vi "Erode_Low_Manual.vi"(4 "Error IN Toolkit":i32, 5 "Error IN LabVIEW":errorcluster, 6 "Radio":i32, 8 "Blocks":i32, 10 "Threads":i32) -> (18 "Error OUT Toolkit":i32, 19 "Error OUT LabVIEW":errorcluster)   [LabVIEW 2018]
doc: "\"Erode\" is the opposite of \"Dilate\". A pixel of the original image (1 or 0) will only be considered 1 if all the pixels that fall behind the kernel window are 1, otherwise it is eroded (zeroed). Therefore, all the pixels near the edges of the objects in the image will be discarded depending on the size of the kernel. It receives the number of threads and blocks for the GPU and the radio known as the kernel, which is the checking area.\n\nFor correct operation it should receive an error that comes from a VI of some processing algorithm or that contains a copy data of CPU-GPU."
uses:
  dll/LibreriaAutis_3.dll
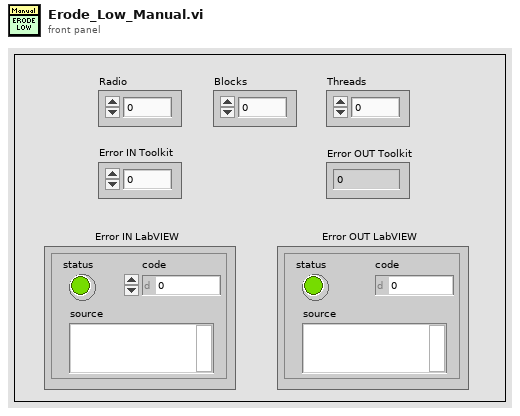
[diagram p1: front panel]
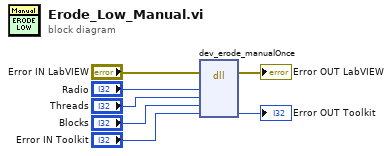
[diagram p0: block diagram]
diagram:
  n1 = dll-call lib="C:/Users/AUTIS/Desktop/LibreriaAUTIS/LabVIEW/dll/LibreriaAutis_3.dll" fn="dev_erode_manualOnce"(error in="Error IN LabVIEW", "radio"="Radio", "threads"="Threads", "blocks"="Blocks", "error"="Error IN Toolkit") -> (error out=→"Error OUT LabVIEW":errorcluster, "error"=→"Error OUT Toolkit":i32)  [unwired: 6 in, 1 out]
